vi "Interpret Driver Controls.vi"() -> ()   [LabVIEW 2018]
uses:
  <vilib>/Rock Robotics/WPI/DriverStation/WPI_DriverStationDerivedRobotMode.ctl
  Robot Global Data.vi
  SubSystems/Controllers/Driver Controller/Driver Controller Global.vi
  SubSystems/Lift/Lift Global.vi
  SubSystems/Drive Train/Drive Train Global.vi
  SubSystems/Controllers/Manipulator Controlller/Manipulator Controller Global.vi
  SubSystems/HAB Climber/HAB Climber Global.vi
  <vilib>/addons/control/pid/pid.llb/PID (DBL).vi
  SubSystems/Cargo Intake/Cargo Intake Global.vi
  SubSystems/Hatch Panel Intake/Hatch Panel Intake Global.vi
  <vilib>/addons/control/pid/NI_PID_pid.lvlib
panel:
  out "Grab Hatch Boolean Thing":bool=TRUE
  in  "Track Scale":dbl
  in  "Last Move Deadband":u32=500
  in  "Last Time Auto":u32=1816077
  in  "Camera Tracking":T1={"proportional gain (Kc)"=0.06, "integral time (Ti, min)"=0.0, "derivative time (Td, min)"=0.0}
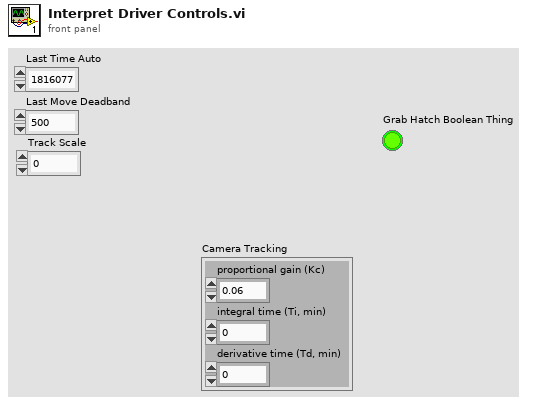
[diagram p1: front panel]
types:
  T1 = cluster{"proportional gain (Kc)":dbl, "integral time (Ti, min)":dbl, "derivative time (Td, min)":dbl}
  T2 = enum16{"Manual", "Hatch Panel Zone 1", "Hatch Panel Zone 2", "Hatch Panel Zone 3", "Cargo Zone 1", "Cargo Zone 2", "Cargo Zone 3", "Cargo Ship Zone"}
  T3 = enum16{"Hatch Panel Zone 1", "Hatch Panel Zone 2", "Hatch Panel Zone 3", "Cargo Zone 1", "Cargo Zone 2", "Cargo Zone 3", "Cargo Ship Zone"}
  T4 = typedef "WPI_DriverStationDerivedRobotMode.ctl" = enum16{"Init", "Execute", "Stop"}
  T5 = cluster{"Rollover":dbl, "Yaw":dbl, "Cont Yaw":dbl}
  T6 = cluster{"offsetAngle H":dbl, "offsetAngle V":dbl, "area":dbl, "skew":dbl, "validTarget":dbl, "latency":dbl}
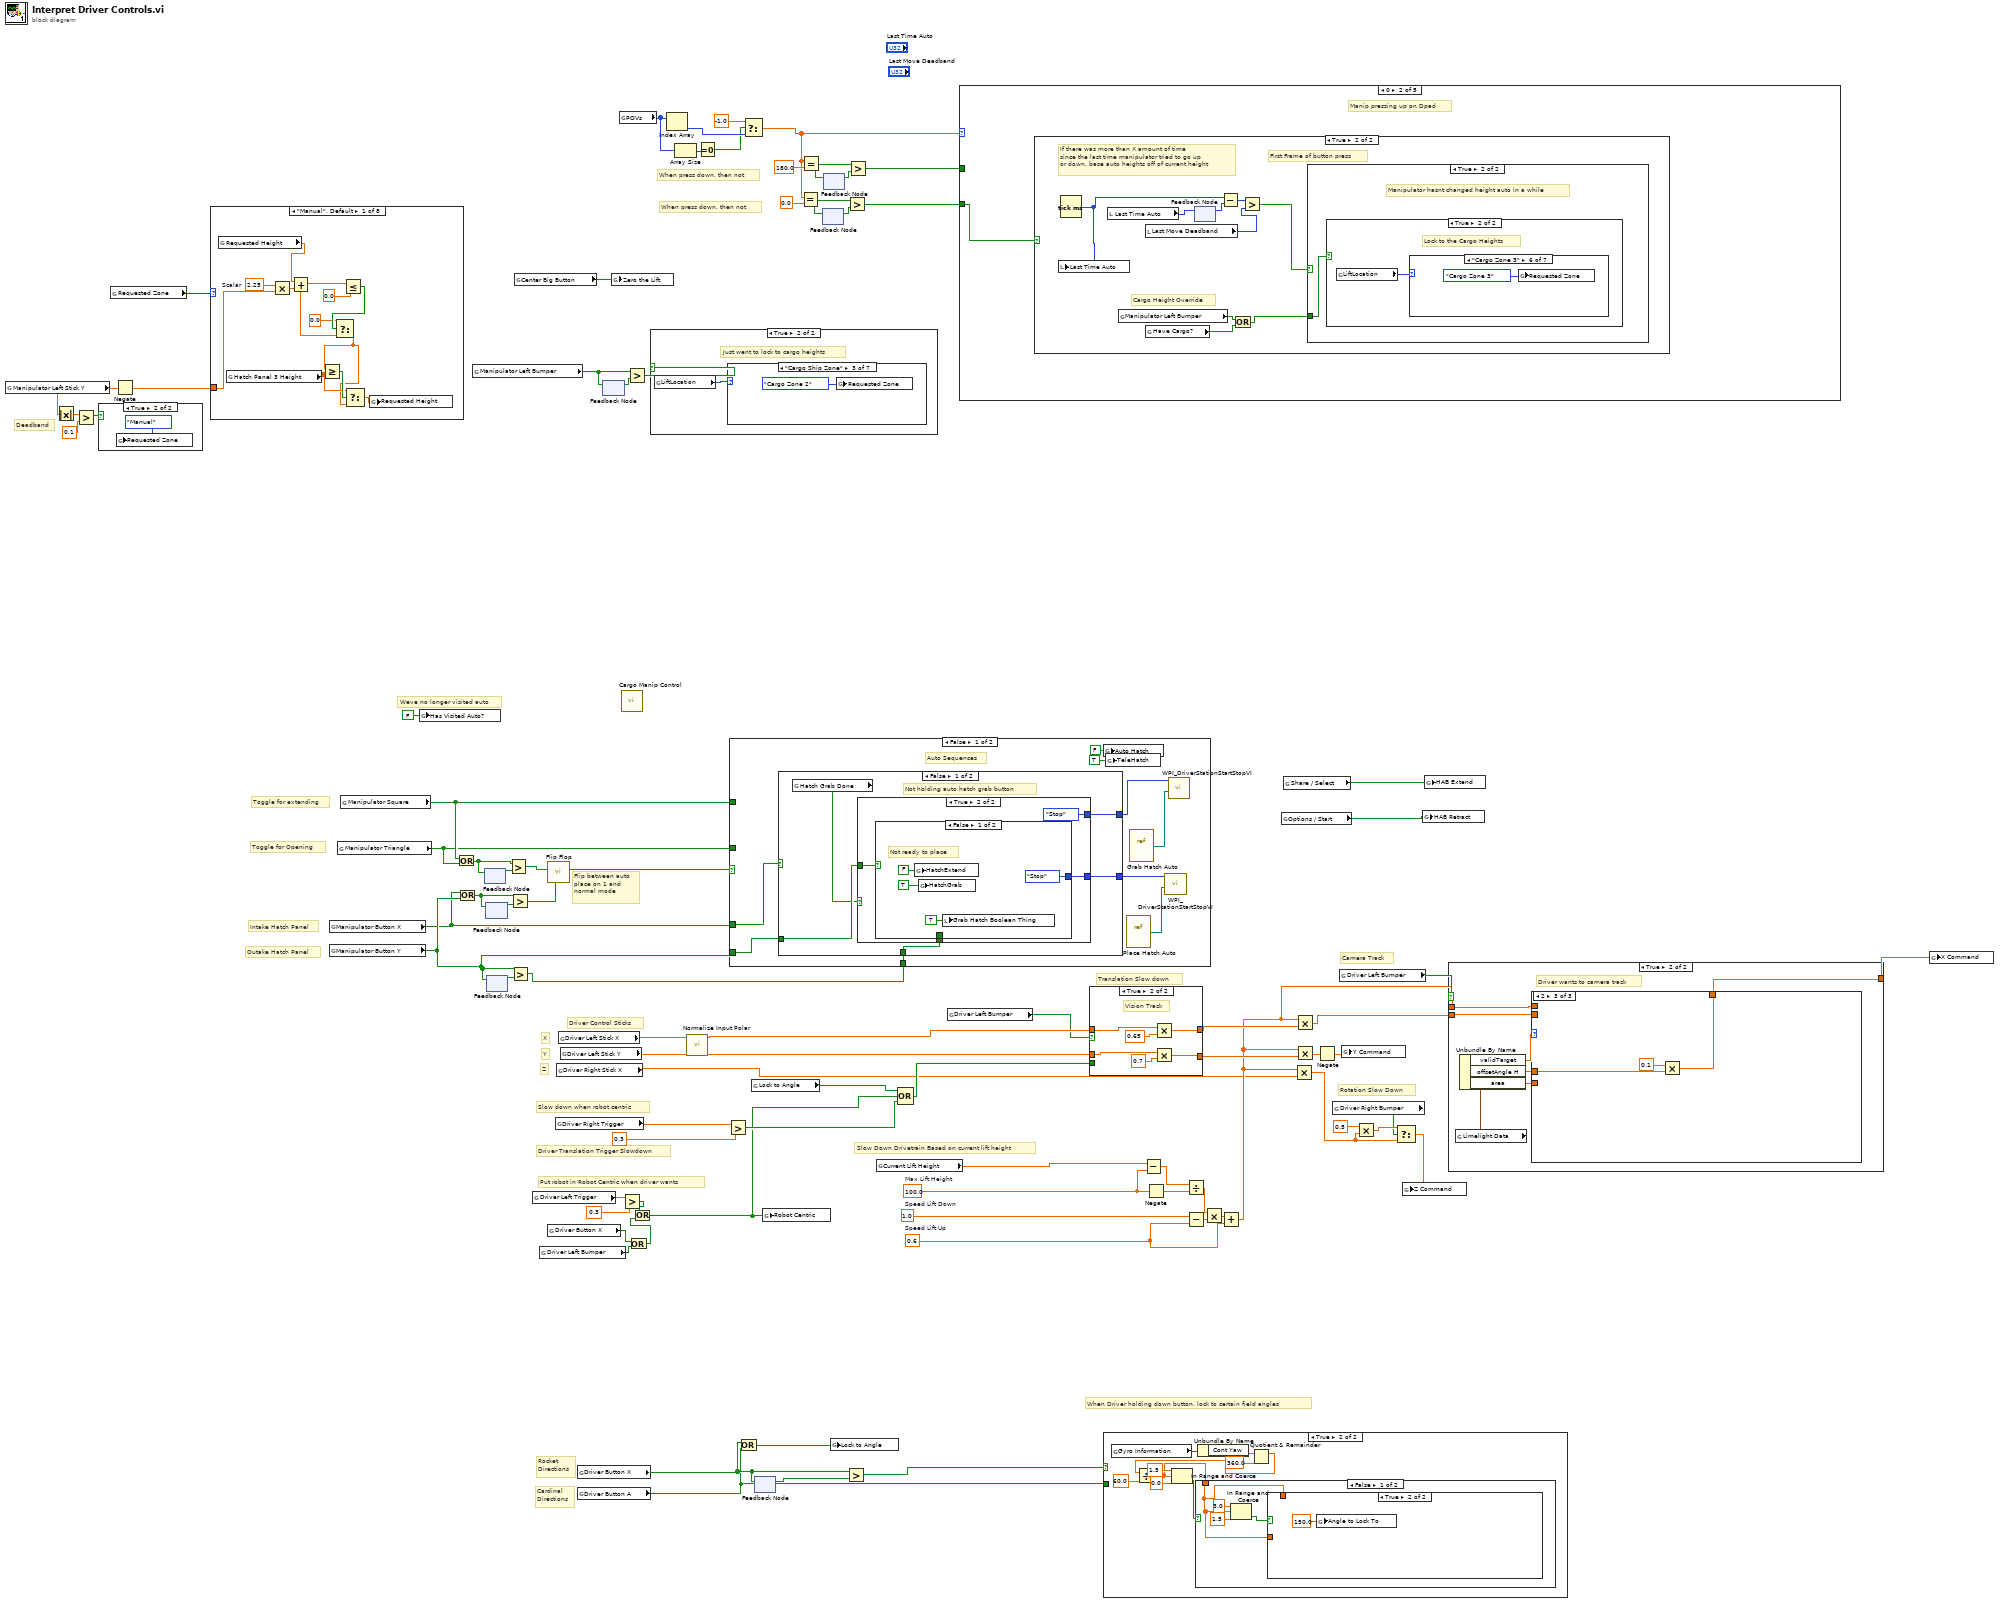
[diagram p0: block diagram]
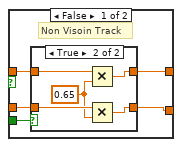
[diagram p2: hidden frame]
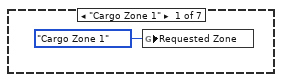
[diagram p5: hidden frame]
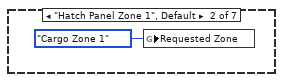
[diagram p6: hidden frame]
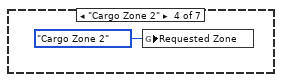
[diagram p7: hidden frame]
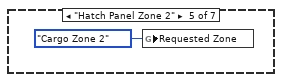
[diagram p8: hidden frame]
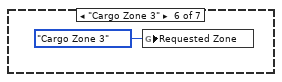
[diagram p9: hidden frame]
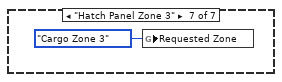
[diagram p10: hidden frame]
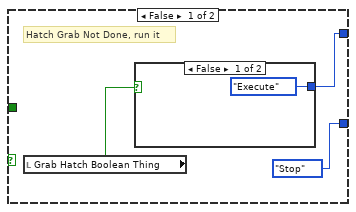
[diagram p11: hidden frame]
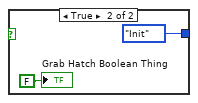
[diagram p12: hidden frame]
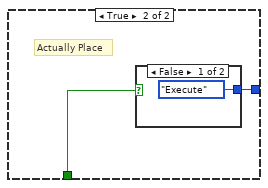
[diagram p13: hidden frame]
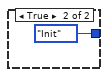
[diagram p14: hidden frame]
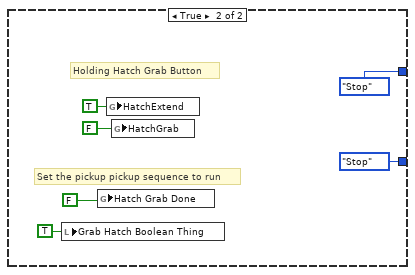
[diagram p15: hidden frame]
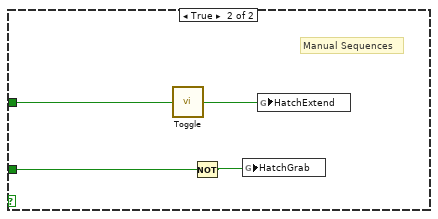
[diagram p16: hidden frame]
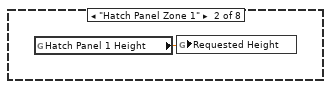
[diagram p18: hidden frame]
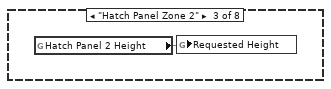
[diagram p19: hidden frame]
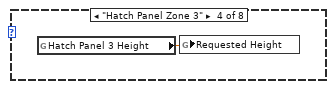
[diagram p20: hidden frame]
diagram:
  w67 = 0.6  # Speed Lift Up
  w71 = 1.0  # Speed Lift Down
  w65 = 100.0  # Max Lift Height
  # "Toggle for Opening"
  # "Toggle for extending"
  # "Outake Hatch Panel"
  # "Intake Hatch Panel"
  # "Flip between auto\nplace on 1 and \nnormal mode"
  # "When press down, then not"
  # "When press down, then not"
  # "Deadband"
  # "Weve no longer visited auto"
  # "Camera Track"
  # "Rotation Slow Down"
  # "Rocket\nDirections"
  # "Cardinal\nDirections"
  # "When Driver holding down button, lock to certain field angles"
  # "Slow Down Drivetrain Based on current lift height"
  # "Put robot in Robot Centric when driver wants"
  # "Slow down when robot centric"
  # "Driver Translation Trigger Slowdown"
  # "Translation Slow down"
  # "Z"
  # "Y"
  # "X"
  # "Driver Control Sticks"
  n1 = global read "Manipulator Controller Global.vi" "Manipulator Left Stick Y"() -> (w40:dbl)
  n2 = Absolute Value(x=w40) -> (abs(x)=w43:dbl)
  n3 = Greater?(x=w43, y=0.1) -> (0:w41:bool)
  n4 = case shown="True" w41 {
    frame False {
    }
    frame True {
      n5 = global write "Lift Global.vi" "Requested Zone"(T2."Manual" ("Requested Zone")) -> ()
    }
  }
  n6 = global read "Lift Global.vi" "Requested Zone"() -> (w44:T2)
  n7 = Negate(x=w40) -> (-x=w39:dbl)
  n8 = case shown="\"Manual\", Default" w44 {
    tunnel: w39 -> [w96 _ _ _ _ _ _ _]
    frame "Manual", Default {
      w95 = 2.25  # Scalar
      n9 = global read "Lift Global.vi" "Requested Height"() -> (w98:dbl)
      n10 = global read "Lift Global.vi" "Hatch Panel 3 Height"() -> (w89:dbl)
      n11 = Multiply(x=w95, y=w96) -> (x*y=w97:dbl)
      n12 = Add(x=w98, y=w97) -> (x+y=w91:dbl)
      n13 = Less Or Equal?(x=w91, y=0.0) -> (x <= y?=w93:bool)
      n14 = Select(t=0.0, s=w93, f=w91) -> (s? t:f=w88:dbl)
      n15 = Greater Or Equal?(x=w88, y=w89) -> (x >= y?=w90:bool)
      n16 = Select(t=w89, s=w90, f=w88) -> (s? t:f=w87:dbl)
      n17 = global write "Lift Global.vi" "Requested Height"(w87) -> ()
    }
    frame "Hatch Panel Zone 1" {
      n18 = global read "Lift Global.vi" "Hatch Panel 1 Height"() -> (w99:dbl)
      n19 = global write "Lift Global.vi" "Requested Height"(w99) -> ()
    }
    frame "Hatch Panel Zone 2" {
      n20 = global read "Lift Global.vi" "Hatch Panel 2 Height"() -> (w100:dbl)
      n21 = global write "Lift Global.vi" "Requested Height"(w100) -> ()
    }
    frame "Hatch Panel Zone 3" {
      n22 = global read "Lift Global.vi" "Hatch Panel 3 Height"() -> (w101:dbl)
      n23 = global write "Lift Global.vi" "Requested Height"(w101) -> ()
    }
    frame "Cargo Zone 1" {
      n24 = global read "Lift Global.vi" "Cargo Zone 1 Height"() -> (w102:dbl)
      n25 = global write "Lift Global.vi" "Requested Height"(w102) -> ()
    }
    frame "Cargo Zone 2" {
      n26 = global read "Lift Global.vi" "Cargo Zone 2 Height"() -> (w103:dbl)
      n27 = global write "Lift Global.vi" "Requested Height"(w103) -> ()
    }
    frame "Cargo Zone 3" {
      n28 = global read "Lift Global.vi" "Cargo Zone 3 Height"() -> (w104:dbl)
      n29 = global write "Lift Global.vi" "Requested Height"(w104) -> ()
    }
    frame "Cargo Ship Zone" {
      n30 = global read "Lift Global.vi" "Cargo Ship Height"() -> (w105:dbl)
      n31 = global write "Lift Global.vi" "Requested Height"(w105) -> ()
    }
  }
  n32 = global read "Manipulator Controller Global.vi" "Manipulator Button X"() -> (w14:bool)
  n33 = global read "Manipulator Controller Global.vi" "Manipulator Button Y"() -> (w16:bool)
  n34 = global read "Manipulator Controller Global.vi" "Manipulator Triangle"() -> (w26:bool)
  n35 = global read "Manipulator Controller Global.vi" "Manipulator Square"() -> (w27:bool)
  n36 = global write "Robot Global Data.vi" "Has Visited Auto?"(FALSE ("Has Visited Auto?")) -> ()
  n37 = Or(x=w27, y=w26) -> (x .or. y?=w24:bool)
  n38 = Or(x=w14, y=w16) -> (x .or. y?=w21:bool)
  n39 = global read "Manipulator Controller Global.vi" "Manipulator Left Bumper"() -> (w12:bool)
  n40 = feedback-in #1(w24) -> ()
  n41 = feedback #1() -> (w25:bool)  [unwired: 1 in]
  n42 = feedback #2() -> (w22:bool)  [unwired: 1 in]
  n43 = feedback-in #2(w21) -> ()
  n44 = feedback #3() -> (w18:bool)  [unwired: 1 in]
  n45 = feedback-in #3(w16) -> ()
  n46 = Greater?(x=w24, y=w25) -> (0:w23:bool)
  n47 = Greater?(x=w21, y=w22) -> (0:w20:bool)
  n48 = Greater?(x=w16, y=w18) -> (0:w17:bool)
  n49 = global read "Manipulator Controller Global.vi" "Center Big Button"() -> (w6:bool)
  n50 = global read "Driver Controller Global.vi" "Driver Left Trigger"() -> (w82:dbl)
  n51 = global read "Driver Controller Global.vi" "Driver Left Bumper"() -> (w3:bool)
  n52 = call "Flip Flop.vi"("Line 2"=w20, "Line 1"=w23) -> ("Switch"=w19:bool)  [unwired: 9 in]
  n53 = global read "Driver Controller Global.vi" "Driver Button X"() -> (w2:bool)
  n54 = global read "Driver Controller Global.vi" "Driver Right Trigger"() -> (w85:dbl)
  n55 = global read "Driver Controller Global.vi" "Driver Right Stick X"() -> (w15:dbl)
  n56 = global read "Driver Controller Global.vi" "Driver Left Stick X"() -> (w8:dbl)
  n57 = global read "Driver Controller Global.vi" "Driver Left Stick Y"() -> (w7:dbl)
  n58 = global read "Driver Controller Global.vi" "Driver Button X"() -> (w63:bool)
  n59 = global read "Driver Controller Global.vi" "Driver Button A"() -> (w61:bool)
  n60 = feedback #4() -> (w13:bool)  [unwired: 1 in]
  n61 = feedback-in #4(w12) -> ()
  n62 = global write "Lift Global.vi" "Zero the Lift"(w6) -> ()
  n63 = global read "Manipulator Controller Global.vi" "POVs"() -> (w48:i16[])
  n64 = call "Cargo Manip Control.vi"() -> ()  [unwired: 12 in]
  n65 = Greater?(x=w82, y=0.3) -> (0:w59:bool)
  n66 = Greater?(x=w12, y=w13) -> (0:w11:bool)
  n67 = Or(x=w2, y=w3) -> (x .or. y?=w1:bool)
  n68 = Or(x=w59, y=w1) -> (x .or. y?=w4:bool)
  n69 = case shown="True" w11 {
    frame False {
    }
    frame True {
      # "Just went to lock to cargo heights"
      n70 = global read "Lift Global.vi" "LiftLocation"() -> (w106:T3)
      n71 = case shown="\"Cargo Ship Zone\"" w106 {
        frame "Cargo Zone 1" {
          n72 = global write "Lift Global.vi" "Requested Zone"(T2."Cargo Zone 1" ("Requested Zone")) -> ()
        }
        frame "Hatch Panel Zone 1", Default {
          n73 = global write "Lift Global.vi" "Requested Zone"(T2."Cargo Zone 1" ("Requested Zone")) -> ()
        }
        frame "Cargo Ship Zone" {
          n74 = global write "Lift Global.vi" "Requested Zone"(T2."Cargo Zone 2" ("Requested Zone")) -> ()
        }
        frame "Cargo Zone 2" {
          n75 = global write "Lift Global.vi" "Requested Zone"(T2."Cargo Zone 2" ("Requested Zone")) -> ()
        }
        frame "Hatch Panel Zone 2" {
          n76 = global write "Lift Global.vi" "Requested Zone"(T2."Cargo Zone 2" ("Requested Zone")) -> ()
        }
        frame "Cargo Zone 3" {
          n77 = global write "Lift Global.vi" "Requested Zone"(T2."Cargo Zone 3" ("Requested Zone")) -> ()
        }
        frame "Hatch Panel Zone 3" {
          n78 = global write "Lift Global.vi" "Requested Zone"(T2."Cargo Zone 3" ("Requested Zone")) -> ()
        }
      }
    }
  }
  n79 = Index Array(array=w48) -> (element=w45:i16)  [unwired: 1 in]
  n80 = Array Size(array=w48) -> (size(s)=w47:i32)
  n81 = call "Normalize Input Polar.vi"("V Input"=w7, "U Input"=w8) -> ("Y Output"=w9:dbl, "X Output"=w10:dbl)  [unwired: 8 in]
  n82 = Equal To 0?(x=w47) -> (x = 0?=w38:bool)
  n83 = Greater?(x=w85, y=0.3) -> (0:w77:bool)
  n84 = case shown="False" w19 {
    tunnel: w26 -> [_ w153]
    tunnel: w27 -> [_ w154]
    tunnel: w14 -> [w122 _]
    tunnel: w17 -> [w119 _]
    tunnel: w16 -> [w118 _]
    frame False {
      # "Auto Sequences"
      n85 = case shown="False" w122 {
        tunnel: [w127 WPI_DriverStationDerivedRobotMode."Stop" ("Call Context")] -> w120
        tunnel: w119 -> [w126 _]
        tunnel: w118 -> [w125 _]
        tunnel: [w123 WPI_DriverStationDerivedRobotMode."Stop" ("Call Context")] -> w116
        frame False {
          # "Not holding auto hatch grab button"
          n86 = global read "Hatch Panel Intake Global.vi" "Hatch Grab Done"() -> (w124:bool)
          n87 = case shown="True" w124 {
            tunnel: [WPI_DriverStationDerivedRobotMode."Stop" ("Call Context") w137] -> w127
            tunnel: w126 -> [_ w136]
            tunnel: w125 -> [_ w135]
            tunnel: [w130 WPI_DriverStationDerivedRobotMode."Stop" ("Call Context")] -> w123
            frame False {
              # "Hatch Grab Not Done, run it"
              n88 = local read "Grab Hatch Boolean Thing"() -> (w128:bool)
              n89 = case shown="False" w128 {
                tunnel: [WPI_DriverStationDerivedRobotMode."Execute" ("Call Context") WPI_DriverStationDerivedRobotMode."Init" ("Call Context")] -> w130
                frame False {
                }
                frame True {
                  "Grab Hatch Boolean Thing" <- FALSE ("Grab Hatch Boolean Thing")
                }
              }
            }
            frame True {
              n90 = case shown="False" w135 {
                tunnel: [WPI_DriverStationDerivedRobotMode."Stop" ("Call Context") w143] -> w137
                tunnel: w136 -> [_ w142]
                frame False {
                  # "Not ready to place"
                  n91 = global write "Hatch Panel Intake Global.vi" "HatchExtend"(FALSE ("HatchExtend")) -> ()
                  n92 = global write "Hatch Panel Intake Global.vi" "HatchGrab"(TRUE ("HatchExtend")) -> ()
                  n93 = local write "Grab Hatch Boolean Thing"(TRUE ("Grab Hatch Boolean Thing")) -> ()
                }
                frame True {
                  # "Actually Place"
                  n94 = case shown="False" w142 {
                    tunnel: [WPI_DriverStationDerivedRobotMode."Execute" ("Call Context") WPI_DriverStationDerivedRobotMode."Init" ("Call Context")] -> w143
                    frame False {
                    }
                    frame True {
                    }
                  }
                }
              }
            }
          }
        }
        frame True {
          # "Set the pickup pickup sequence to run"
          # "Holding Hatch Grab Button"
          n95 = local write "Grab Hatch Boolean Thing"(TRUE ("Grab Hatch Boolean Thing")) -> ()
          n96 = global write "Hatch Panel Intake Global.vi" "Hatch Grab Done"(FALSE ("HatchExtend")) -> ()
          n97 = global write "Hatch Panel Intake Global.vi" "HatchExtend"(TRUE ("HatchExtend")) -> ()
          n98 = global write "Hatch Panel Intake Global.vi" "HatchGrab"(FALSE ("HatchExtend")) -> ()
        }
      }
      n99 = global write "Hatch Panel Intake Global.vi" "Auto Hatch"(FALSE ("TeleHatch")) -> ()
      n100 = global write "Hatch Panel Intake Global.vi" "TeleHatch"(TRUE ("TeleHatch")) -> ()
      n101 = vi-ref "Place Hatch Auto.vi"() -> (w121:refnum<vi>)
      n102 = vi-ref "Grab Hatch Auto.vi"() -> (w117:refnum<vi>)
      n103 = call <vilib>:"WPI_DriverStationStartStopVI.vi"("VI in"=w121, "Call Context"=w120) -> ()  [unwired: 10 in]
      n104 = call <vilib>:"WPI_DriverStationStartStopVI.vi"("VI in"=w117, "Call Context"=w116) -> ()  [unwired: 10 in]
    }
    frame True {
      # "Manual Sequences"
      n105 = call "Toggle.vi"("Input"=w154) -> ("Output"=w155:bool)
      n106 = Not(x=w153) -> (.not. x?=w152:bool)
      n107 = global write "Hatch Panel Intake Global.vi" "HatchGrab"(w152) -> ()
      n108 = global write "Hatch Panel Intake Global.vi" "HatchExtend"(w155) -> ()
    }
  }
  n109 = Or(x=w63, y=w61) -> (x .or. y?=w60:bool)
  n110 = Select(t=-1.0, s=w38, f=w45) -> (s? t:f=w30:dbl)
  n111 = global read "Drive Train Global.vi" "Lock to Angle"() -> (w58:bool)
  n112 = feedback #5() -> (w64:bool)  [unwired: 1 in]
  n113 = feedback-in #5(w63) -> ()
  n114 = global write "Drive Train Global.vi" "Robot Centric"(w4) -> ()
  n115 = Equal?(x=w30, y=0.0) -> (x = y?=w33:bool)
  n116 = Equal?(x=w30, y=180.0) -> (x = y?=w35:bool)
  n117 = feedback #6() -> (w32:bool)  [unwired: 1 in]
  n118 = feedback-in #6(w33) -> ()
  n119 = feedback-in #7(w35) -> ()
  n120 = feedback #7() -> (w36:bool)  [unwired: 1 in]
  n121 = global write "Drive Train Global.vi" "Lock to Angle"(w60) -> ()
  n122 = Greater?(x=w63, y=w64) -> (0:w62:bool)
  n123 = Greater?(x=w33, y=w32) -> (0:w29:bool)
  n124 = Greater?(x=w35, y=w36) -> (0:w34:bool)
  n125 = global read "Lift Global.vi" "Current Lift Height"() -> (w73:dbl)
  n126 = Compound Arithmetic op=OR(w58, w4, w77) -> (w76:bool)
  n127 = global read "Driver Controller Global.vi" "Driver Left Bumper"() -> (w5:bool)
  n128 = case shown="0" w30 {
    tunnel: w34 -> [_ _ w200 _ _]
    tunnel: w29 -> [_ w156 _ _ _]
    frame -1, Default {
      # "Nothing on the D-Pad is pressed!"
    }
    frame 0 {
      # "Manip pressing up on Dpad"
      n129 = case shown="True" w156 {
        frame False {
          # "Still pressing button, do nothing"
        }
        frame True {
          # "Cargo Height Override"
          # "First Frame of button press"
          # "If there was more than X amount of time\nsince the last time manipulator tried to go up\nor down, base auto heights off of current height"
          n130 = Tick Count (ms)() -> (millisecond timer value=w162:u32)
          n131 = local write "Last Time Auto"(w162) -> ()
          n132 = local read "Last Time Auto"() -> (w161:u32)
          n133 = global read "Manipulator Controller Global.vi" "Manipulator Left Bumper"() -> (w159:bool)
          n134 = local read "Last Move Deadband"() -> (w163:u32)
          n135 = global read "Cargo Intake Global.vi" "Have Cargo?"() -> (w157:bool)
          n136 = feedback #8() -> (w160:u32)  [unwired: 1 in]
          n137 = feedback-in #8(w161) -> ()
          n138 = Subtract(x=w162, y=w160) -> (x-y=w165:u32)
          n139 = Or(x=w159, y=w157) -> (x .or. y?=w158:bool)
          n140 = Greater?(x=w165, y=w163) -> (0:w164:bool)
          n141 = case shown="True" w164 {
            tunnel: w158 -> [w166 w183]
            frame False {
              # "Manipulator is still changing height to go to"
              n142 = case shown="False" w166 {
                frame False {
                  # "Lock to the Hatch Heights"
                  n143 = global read "Lift Global.vi" "Requested Zone"() -> (w167:T2)
                  n144 = case shown="\"Hatch Panel Zone 3\"" w167 {
                    frame "Manual" {
                    }
                    frame "Cargo Zone 1" {
                      n145 = global write "Lift Global.vi" "Requested Zone"(T2."Hatch Panel Zone 1" ("Requested Zone")) -> ()
                    }
                    frame "Hatch Panel Zone 1", Default {
                      n146 = global write "Lift Global.vi" "Requested Zone"(T2."Hatch Panel Zone 2" ("Requested Zone")) -> ()
                    }
                    frame "Cargo Ship Zone" {
                      n147 = global write "Lift Global.vi" "Requested Zone"(T2."Hatch Panel Zone 2" ("Requested Zone")) -> ()
                    }
                    frame "Cargo Zone 2" {
                      n148 = global write "Lift Global.vi" "Requested Zone"(T2."Hatch Panel Zone 2" ("Requested Zone")) -> ()
                    }
                    frame "Hatch Panel Zone 2" {
                      n149 = global write "Lift Global.vi" "Requested Zone"(T2."Hatch Panel Zone 3" ("Requested Zone")) -> ()
                    }
                    frame "Cargo Zone 3" {
                      n150 = global write "Lift Global.vi" "Requested Zone"(T2."Hatch Panel Zone 3" ("Requested Zone")) -> ()
                    }
                    frame "Hatch Panel Zone 3" {
                      n151 = global write "Lift Global.vi" "Requested Zone"(T2."Hatch Panel Zone 3" ("Requested Zone")) -> ()
                    }
                  }
                }
                frame True {
                  # "Lock to the Cargo Heights"
                  n152 = global read "Lift Global.vi" "Requested Zone"() -> (w175:T2)
                  n153 = case shown="\"Manual\"" w175 {
                    frame "Manual" {
                    }
                    frame "Cargo Zone 1" {
                      n154 = global write "Lift Global.vi" "Requested Zone"(T2."Cargo Zone 2" ("Requested Zone")) -> ()
                    }
                    frame "Hatch Panel Zone 1", Default {
                      n155 = global write "Lift Global.vi" "Requested Zone"(T2."Cargo Zone 2" ("Requested Zone")) -> ()
                    }
                    frame "Cargo Ship Zone" {
                      n156 = global write "Lift Global.vi" "Requested Zone"(T2."Cargo Zone 2" ("Requested Zone")) -> ()
                    }
                    frame "Cargo Zone 2" {
                      n157 = global write "Lift Global.vi" "Requested Zone"(T2."Cargo Zone 3" ("Requested Zone")) -> ()
                    }
                    frame "Hatch Panel Zone 2" {
                      n158 = global write "Lift Global.vi" "Requested Zone"(T2."Cargo Zone 3" ("Requested Zone")) -> ()
                    }
                    frame "Cargo Zone 3" {
                      n159 = global write "Lift Global.vi" "Requested Zone"(T2."Cargo Zone 3" ("Requested Zone")) -> ()
                    }
                    frame "Hatch Panel Zone 3" {
                      n160 = global write "Lift Global.vi" "Requested Zone"(T2."Cargo Zone 3" ("Requested Zone")) -> ()
                    }
                  }
                }
              }
            }
            frame True {
              # "Manipulator hasnt changed height auto in a while"
              n161 = case shown="True" w183 {
                frame False {
                  # "Lock to the Hatch Heights"
                  n162 = global read "Lift Global.vi" "LiftLocation"() -> (w184:T3)
                  n163 = case shown="\"Cargo Zone 1\"" w184 {
                    frame "Cargo Zone 1" {
                      n164 = global write "Lift Global.vi" "Requested Zone"(T2."Hatch Panel Zone 1" ("Requested Zone")) -> ()
                    }
                    frame "Hatch Panel Zone 1", Default {
                      n165 = global write "Lift Global.vi" "Requested Zone"(T2."Hatch Panel Zone 2" ("Requested Zone")) -> ()
                    }
                    frame "Cargo Ship Zone" {
                      n166 = global write "Lift Global.vi" "Requested Zone"(T2."Hatch Panel Zone 2" ("Requested Zone")) -> ()
                    }
                    frame "Cargo Zone 2" {
                      n167 = global write "Lift Global.vi" "Requested Zone"(T2."Hatch Panel Zone 2" ("Requested Zone")) -> ()
                    }
                    frame "Hatch Panel Zone 2" {
                      n168 = global write "Lift Global.vi" "Requested Zone"(T2."Hatch Panel Zone 3" ("Requested Zone")) -> ()
                    }
                    frame "Cargo Zone 3" {
                      n169 = global write "Lift Global.vi" "Requested Zone"(T2."Hatch Panel Zone 3" ("Requested Zone")) -> ()
                    }
                    frame "Hatch Panel Zone 3" {
                      n170 = global write "Lift Global.vi" "Requested Zone"(T2."Hatch Panel Zone 3" ("Requested Zone")) -> ()
                    }
                  }
                }
                frame True {
                  # "Lock to the Cargo Heights"
                  n171 = global read "Lift Global.vi" "LiftLocation"() -> (w192:T3)
                  n172 = case shown="\"Cargo Zone 3\"" w192 {
                    frame "Cargo Zone 1" {
                      n173 = global write "Lift Global.vi" "Requested Zone"(T2."Cargo Zone 2" ("Requested Zone")) -> ()
                    }
                    frame "Hatch Panel Zone 1", Default {
                      n174 = global write "Lift Global.vi" "Requested Zone"(T2."Cargo Zone 2" ("Requested Zone")) -> ()
                    }
                    frame "Cargo Ship Zone" {
                      n175 = global write "Lift Global.vi" "Requested Zone"(T2."Cargo Zone 2" ("Requested Zone")) -> ()
                    }
                    frame "Cargo Zone 2" {
                      n176 = global write "Lift Global.vi" "Requested Zone"(T2."Cargo Zone 3" ("Requested Zone")) -> ()
                    }
                    frame "Hatch Panel Zone 2" {
                      n177 = global write "Lift Global.vi" "Requested Zone"(T2."Cargo Zone 3" ("Requested Zone")) -> ()
                    }
                    frame "Cargo Zone 3" {
                      n178 = global write "Lift Global.vi" "Requested Zone"(T2."Cargo Zone 3" ("Requested Zone")) -> ()
                    }
                    frame "Hatch Panel Zone 3" {
                      n179 = global write "Lift Global.vi" "Requested Zone"(T2."Cargo Zone 3" ("Requested Zone")) -> ()
                    }
                  }
                }
              }
            }
          }
        }
      }
    }
    frame 180 {
      # "Manip pressing down on Dpad"
      n180 = case shown="True" w200 {
        frame False {
          # "Still pressing button, do nothing"
        }
        frame True {
          # "Cargo Height Override"
          # "First frame of button press"
          # "If there was more than X amount of time\nsince the last time manipulator tried to go up\nor down, base auto heights off of current height"
          n181 = Tick Count (ms)() -> (millisecond timer value=w208:u32)
          n182 = local write "Last Time Auto"(w208) -> ()
          n183 = local read "Last Time Auto"() -> (w206:u32)
          n184 = global read "Manipulator Controller Global.vi" "Manipulator Left Bumper"() -> (w203:bool)
          n185 = local read "Last Move Deadband"() -> (w207:u32)
          n186 = global read "Cargo Intake Global.vi" "Have Cargo?"() -> (w202:bool)
          n187 = feedback #9() -> (w205:u32)  [unwired: 1 in]
          n188 = feedback-in #9(w206) -> ()
          n189 = Subtract(x=w208, y=w205) -> (x-y=w209:u32)
          n190 = Greater?(x=w209, y=w207) -> (0:w204:bool)
          n191 = Or(x=w203, y=w202) -> (x .or. y?=w201:bool)
          n192 = case shown="False" w204 {
            tunnel: w201 -> [w210 w227]
            frame False {
              # "Manipulator is still changing height to go to"
              n193 = case shown="False" w210 {
                frame False {
                  # "Lock to the Hatch Heights"
                  n194 = global read "Lift Global.vi" "Requested Zone"() -> (w211:T2)
                  n195 = case shown="\"Hatch Panel Zone 3\"" w211 {
                    frame "Manual" {
                    }
                    frame "Cargo Zone 1" {
                      n196 = global write "Lift Global.vi" "Requested Zone"(T2."Hatch Panel Zone 1" ("Requested Zone")) -> ()
                    }
                    frame "Hatch Panel Zone 1", Default {
                      n197 = global write "Lift Global.vi" "Requested Zone"(T2."Hatch Panel Zone 1" ("Requested Zone")) -> ()
                    }
                    frame "Cargo Ship Zone" {
                      n198 = global write "Lift Global.vi" "Requested Zone"(T2."Hatch Panel Zone 1" ("Requested Zone")) -> ()
                    }
                    frame "Cargo Zone 2" {
                      n199 = global write "Lift Global.vi" "Requested Zone"(T2."Hatch Panel Zone 1" ("Requested Zone")) -> ()
                    }
                    frame "Hatch Panel Zone 2" {
                      n200 = global write "Lift Global.vi" "Requested Zone"(T2."Hatch Panel Zone 1" ("Requested Zone")) -> ()
                    }
                    frame "Cargo Zone 3" {
                      n201 = global write "Lift Global.vi" "Requested Zone"(T2."Hatch Panel Zone 2" ("Requested Zone")) -> ()
                    }
                    frame "Hatch Panel Zone 3" {
                      n202 = global write "Lift Global.vi" "Requested Zone"(T2."Hatch Panel Zone 2" ("Requested Zone")) -> ()
                    }
                  }
                }
                frame True {
                  # "Lock to the Cargo Heights"
                  n203 = global read "Lift Global.vi" "Requested Zone"() -> (w219:T2)
                  n204 = case shown="\"Manual\"" w219 {
                    frame "Manual" {
                    }
                    frame "Cargo Zone 1" {
                      n205 = global write "Lift Global.vi" "Requested Zone"(T2."Cargo Zone 1" ("Requested Zone")) -> ()
                    }
                    frame "Hatch Panel Zone 1", Default {
                      n206 = global write "Lift Global.vi" "Requested Zone"(T2."Cargo Zone 1" ("Requested Zone")) -> ()
                    }
                    frame "Cargo Ship Zone" {
                      n207 = global write "Lift Global.vi" "Requested Zone"(T2."Cargo Zone 1" ("Requested Zone")) -> ()
                    }
                    frame "Cargo Zone 2" {
                      n208 = global write "Lift Global.vi" "Requested Zone"(T2."Cargo Zone 1" ("Requested Zone")) -> ()
                    }
                    frame "Hatch Panel Zone 2" {
                      n209 = global write "Lift Global.vi" "Requested Zone"(T2."Cargo Zone 2" ("Requested Zone")) -> ()
                    }
                    frame "Cargo Zone 3" {
                      n210 = global write "Lift Global.vi" "Requested Zone"(T2."Cargo Zone 2" ("Requested Zone")) -> ()
                    }
                    frame "Hatch Panel Zone 3" {
                      n211 = global write "Lift Global.vi" "Requested Zone"(T2."Cargo Zone 3" ("Requested Zone")) -> ()
                    }
                  }
                }
              }
            }
            frame True {
              # "Manipulator hasnt changed height auto in a while"
              n212 = case shown="False" w227 {
                frame False {
                  # "Lock to the Hatch Heights"
                  n213 = global read "Lift Global.vi" "LiftLocation"() -> (w228:T3)
                  n214 = case shown="\"Hatch Panel Zone 3\"" w228 {
                    frame "Cargo Zone 1" {
                      n215 = global write "Lift Global.vi" "Requested Zone"(T2."Hatch Panel Zone 1" ("Requested Zone")) -> ()
                    }
                    frame "Hatch Panel Zone 1", Default {
                      n216 = global write "Lift Global.vi" "Requested Zone"(T2."Hatch Panel Zone 1" ("Requested Zone")) -> ()
                    }
                    frame "Cargo Ship Zone" {
                      n217 = global write "Lift Global.vi" "Requested Zone"(T2."Hatch Panel Zone 1" ("Requested Zone")) -> ()
                    }
                    frame "Cargo Zone 2" {
                      n218 = global write "Lift Global.vi" "Requested Zone"(T2."Hatch Panel Zone 1" ("Requested Zone")) -> ()
                    }
                    frame "Hatch Panel Zone 2" {
                      n219 = global write "Lift Global.vi" "Requested Zone"(T2."Hatch Panel Zone 1" ("Requested Zone")) -> ()
                    }
                    frame "Cargo Zone 3" {
                      n220 = global write "Lift Global.vi" "Requested Zone"(T2."Hatch Panel Zone 2" ("Requested Zone")) -> ()
                    }
                    frame "Hatch Panel Zone 3" {
                      n221 = global write "Lift Global.vi" "Requested Zone"(T2."Hatch Panel Zone 2" ("Requested Zone")) -> ()
                    }
                  }
                }
                frame True {
                  # "Lock to the Cargo Heights"
                  n222 = global read "Lift Global.vi" "LiftLocation"() -> (w236:T3)
                  n223 = case shown="\"Hatch Panel Zone 3\"" w236 {
                    frame "Cargo Zone 1" {
                      n224 = global write "Lift Global.vi" "Requested Zone"(T2."Cargo Zone 1" ("Requested Zone")) -> ()
                    }
                    frame "Hatch Panel Zone 1", Default {
                      n225 = global write "Lift Global.vi" "Requested Zone"(T2."Cargo Zone 1" ("Requested Zone")) -> ()
                    }
                    frame "Cargo Ship Zone" {
                      n226 = global write "Lift Global.vi" "Requested Zone"(T2."Cargo Zone 1" ("Requested Zone")) -> ()
                    }
                    frame "Cargo Zone 2" {
                      n227 = global write "Lift Global.vi" "Requested Zone"(T2."Cargo Zone 1" ("Requested Zone")) -> ()
                    }
                    frame "Hatch Panel Zone 2" {
                      n228 = global write "Lift Global.vi" "Requested Zone"(T2."Cargo Zone 2" ("Requested Zone")) -> ()
                    }
                    frame "Cargo Zone 3" {
                      n229 = global write "Lift Global.vi" "Requested Zone"(T2."Cargo Zone 2" ("Requested Zone")) -> ()
                    }
                    frame "Hatch Panel Zone 3" {
                      n230 = global write "Lift Global.vi" "Requested Zone"(T2."Cargo Zone 3" ("Requested Zone")) -> ()
                    }
                  }
                }
              }
            }
          }
        }
      }
    }
    frame 90 {
      # "Go to Cargo in Cargo Ship Height"
      # "Right on D-Pad"
      n231 = global write "Lift Global.vi" "Requested Zone"(T2."Cargo Ship Zone" ("Requested Zone")) -> ()
    }
    frame 270 {
      # "Go to Hatch Level 1 Height"
      # "Left on D-Pad"
      n232 = global write "Lift Global.vi" "Requested Zone"(T2."Hatch Panel Zone 1" ("Requested Zone")) -> ()
    }
  }
  n233 = case shown="True" w5 {
    tunnel: w76 -> [w250 _]
    tunnel: [w249 w262] -> w75
    tunnel: [w248 w263] -> w74
    tunnel: w10 -> [w247 w260]
    tunnel: w9 -> [w246 w261]
    frame False {
      # "Non Visoin Track"
      n234 = case shown="True" w250 {
        tunnel: w246 -> [w252 w257]
        tunnel: [w252 w256] -> w249
        tunnel: [w251 w255] -> w248
        tunnel: w247 -> [w251 w254]
        frame False {
        }
        frame True {
          w253 = 0.65 ("Y Slower")
          n235 = Multiply(x=w254, y=w253) -> (x*y=w255:dbl)
          n236 = Multiply(x=w257, y=w253) -> (x*y=w256:dbl)
        }
      }
    }
    frame True {
      # "Vision Track"
      n237 = Multiply(x=w260, y=0.65 ("Y Slower")) -> (x*y=w263:dbl)
      n238 = Multiply(x=w261, y=0.7 ("Y Slower")) -> (x*y=w262:dbl)
    }
  }
  n239 = case shown="True" w62 {
    tunnel: w61 -> [w265 _]
    frame False {
      n240 = feedback #10() -> (w266:bool)  [unwired: 1 in]
      n241 = feedback-in #10(w265) -> ()
      n242 = Greater?(x=w265, y=w266) -> (0:w264:bool)
      n243 = case shown="True" w264 {
        frame False {
        }
        frame True {
          n244 = global read "Drive Train Global.vi" "Gyro Information"() -> (w273:T5)
          n245 = Unbundle By Name(w273) -> ("Yaw"=w270:dbl)
          n246 = Add(x=w270, y=180.0) -> (x+y=w269:dbl)
          n247 = Divide(x=w269, y=90.0) -> (x/y=w271:dbl)
          n248 = Round To Nearest(number=w271) -> (nearest integer value=w267:dbl)
          n249 = case shown="1" w267 {
            frame 0, Default {
              n250 = global write "Drive Train Global.vi" "Angle to Lock To"(180.0 ("Angle to Lock To")) -> ()
            }
            frame 1 {
              n251 = global write "Drive Train Global.vi" "Angle to Lock To"(270.0 ("Angle to Lock To")) -> ()
            }
            frame 2 {
              n252 = global write "Drive Train Global.vi" "Angle to Lock To"(0.0 ("Angle to Lock To")) -> ()
            }
            frame 3 {
              n253 = global write "Drive Train Global.vi" "Angle to Lock To"(90.0 ("Angle to Lock To")) -> ()
            }
            frame 4 {
              n254 = global write "Drive Train Global.vi" "Angle to Lock To"(180.0 ("Angle to Lock To")) -> ()
            }
          }
        }
      }
    }
    frame True {
      n255 = global read "Drive Train Global.vi" "Gyro Information"() -> (w287:T5)
      n256 = Unbundle By Name(w287) -> ("Cont Yaw"=w285:dbl)
      n257 = Quotient & Remainder(x=w285, y=360.0) -> (x-y*floor(x/y)=w283:dbl)  [unwired: 1 out]
      n258 = Divide(x=w283, y=60.0) -> (x/y=w279:dbl)
      n259 = In Range and Coerce(upper limit=1.5, x=w279, lower limit=0.0) -> (In Range?=w280:bool)  [unwired: 1 out]
      n260 = case shown="False" w280 {
        tunnel: w279 -> [w288 _]
        frame False {
          n261 = In Range and Coerce(upper limit=3.0, x=w288, lower limit=1.5) -> (In Range?=w289:bool)  [unwired: 1 out]
          n262 = case shown="True" w289 {
            tunnel: w288 -> [w294 _]
            tunnel: w288 -> [w292 _]
            frame False {
              n263 = In Range and Coerce(upper limit=4.5, x=w294, lower limit=3.0) -> (In Range?=w293:bool)  [unwired: 1 out]
              n264 = case shown="False" w293 {
                tunnel: w292 -> [w298 _]
                frame False {
                  n265 = In Range and Coerce(upper limit=6.0, x=w298, lower limit=4.5) -> (In Range?=w297:bool)  [unwired: 1 out]
                  n266 = case shown="True" w297 {
                    frame False {
                    }
                    frame True {
                      n267 = global write "Drive Train Global.vi" "Angle to Lock To"(330.0 ("Angle to Lock To")) -> ()
                    }
                  }
                }
                frame True {
                  n268 = global write "Drive Train Global.vi" "Angle to Lock To"(210.0 ("Angle to Lock To")) -> ()
                }
              }
            }
            frame True {
              n269 = global write "Drive Train Global.vi" "Angle to Lock To"(150.0 ("Angle to Lock To")) -> ()
            }
          }
        }
        frame True {
          n270 = global write "Drive Train Global.vi" "Angle to Lock To"(30.0 ("Angle to Lock To")) -> ()
        }
      }
    }
  }
  n271 = Subtract(x=w73, y=w65) -> (x-y=w72:dbl)
  n272 = Negate(x=w65) -> (-x=w66:dbl)
  n273 = Divide(x=w72, y=w66) -> (x/y=w70:dbl)
  n274 = Subtract(x=w71, y=w67) -> (x-y=w69:dbl)
  n275 = Multiply(x=w70, y=w69) -> (x*y=w68:dbl)
  n276 = Add(x=w68, y=w67) -> (x+y=w28:dbl)
  n277 = global read "Manipulator Controller Global.vi" "Options / Start"() -> (w52:bool)
  n278 = global read "Manipulator Controller Global.vi" "Share / Select"() -> (w53:bool)
  n279 = Multiply(x=w28, y=w15) -> (x*y=w81:dbl)
  n280 = Multiply(x=w28, y=w74) -> (x*y=w55:dbl)
  n281 = Multiply(x=w28, y=w75) -> (x*y=w51:dbl)
  n282 = Negate(x=w51) -> (-x=w50:dbl)
  n283 = global read "Driver Controller Global.vi" "Driver Right Bumper"() -> (w78:bool)
  n284 = global read "Driver Controller Global.vi" "Driver Left Bumper"() -> (w57:bool)
  n285 = global write "Drive Train Global.vi" "Y Command"(w50) -> ()
  n286 = Multiply(x=0.5, y=w81) -> (x*y=w80:dbl)
  n287 = Select(t=w80, s=w78, f=w81) -> (s? t:f=w56:dbl)
  n288 = global write "Drive Train Global.vi" "Z Command"(w56) -> ()
  n289 = global write "HAB Climber Global.vi" "HAB Retract"(w52) -> ()
  n290 = global write "HAB Climber Global.vi" "HAB Extend"(w53) -> ()
  n291 = case shown="True" w57 {
    tunnel: w55 -> [w306 w311]
    tunnel: [w306 w309] -> w54
    tunnel: w28 -> [_ w308]
    frame False {
      # "Driver not attepting to camera track, be normal"
      n292 = global write "Driver Controller Global.vi" "Output On"(FALSE ("Rumble Controller?")) -> ()
    }
    frame True {
      # "Driver wants to camera track"
      n293 = global read "Robot Global Data.vi" "Limelight Data"() -> (w313:T6)
      n294 = Unbundle By Name(w313) -> ("validTarget"=w312:dbl, "offsetAngle H"=w310:dbl, "area"=w307:dbl)
      n295 = case shown="2" w312 {
        tunnel: w311 -> [w316 _ _]
        tunnel: w310 -> [_ w335 w339]
        tunnel: [w316 w334 w340] -> w309
        tunnel: w308 -> [_ w332 _]
        tunnel: w307 -> [_ w327 _]
        frame 0, Default {
          # "No Valid Target, keep using driver controls\nand rumble controller so knows not tracking"
          n296 = global write "Driver Controller Global.vi" "Rumble Right"(1.0 ("Rumble Amount")) -> ()
          n297 = global write "Driver Controller Global.vi" "Rumble Left"(1.0 ("Rumble Amount")) -> ()
          n298 = global write "Driver Controller Global.vi" "Output On"(TRUE ("Rumble Controller?")) -> ()
        }
        frame 1 {
          # "There is a valid target, track target"
          n299 = Reciprocal(x=w327) -> (1/x=w326:dbl)
          n300 = Unbundle By Name("Camera Tracking") -> ("proportional gain (Kc)"=w320:dbl, "integral time (Ti, min)"=w330:dbl, "derivative time (Td, min)"=w329:dbl)
          n301 = Multiply(x=w326, y="Track Scale") -> (x*y=w319:dbl)
          n302 = Subtract(x=1.0, y="Track Scale") -> (x-y=w323:dbl)
          n303 = Multiply(x=w319, y=w320) -> (x*y=w318:dbl)
          n304 = Multiply(x=w320, y=w323) -> (x*y=w322:dbl)
          n305 = Add(x=w318, y=w322) -> (x+y=w321:dbl)
          n306 = Bundle By Name(cluster="Camera Tracking", "proportional gain (Kc)"=w321, "integral time (Ti, min)"=w330, "derivative time (Td, min)"=w329) -> (w328:T1)
          n307 = call-poly <vilib>:"PID.vi"("output range"=cluster{"output high":dbl, "output low":dbl} {"output high"=1.0, "output low"=-1.0}, "PID gains"=w328, "setpoint"=w335) -> ("output"=w333:dbl)  [unwired: 7 in, 1 out]
          n308 = Multiply(x=w332, y=w333) -> (x*y=w334:dbl)
          n309 = global write "Driver Controller Global.vi" "Output On"(FALSE ("Rumble Controller?")) -> ()
        }
        frame 2 {
          n310 = Multiply(x=0.1, y=w339) -> (x*y=w340:dbl)
        }
      }
    }
  }
  n311 = global write "Drive Train Global.vi" "X Command"(w54) -> ()
